vi "Initialize State Variables.vi"(8 "error in":errorcluster) -> (0 "error out":errorcluster, 2 "State Vars":T1)   [LabVIEW 2014, in "Waveform-Processing-Custom-Device Engine.lvlib"]
uses:
  Waveform-Processing-Custom-Device Engine.lvlib
  Types/StateVars.ctl
  Types/Async FIFOs.ctl
  Types/Async Settings.ctl
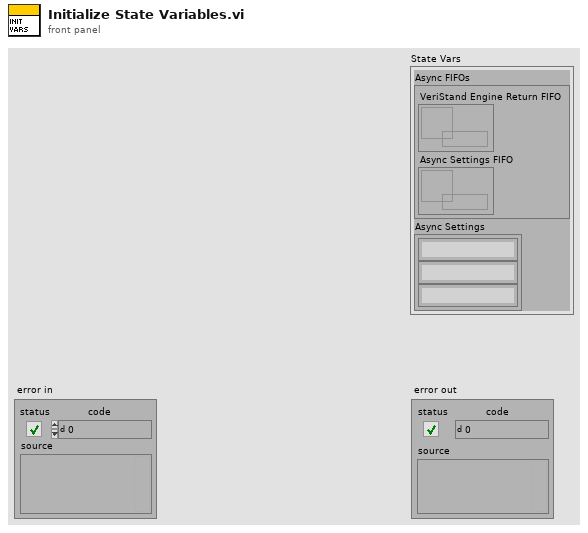
[diagram p1: front panel]
types:
  T1 = typedef "Waveform-Processing-Custom-Device Engine.lvlib/StateVars.ctl" = cluster{"Async FIFOs":T2, "Async Settings":T3}
  T2 = typedef "Async FIFOs.ctl" = cluster{"VeriStand Engine Return FIFO":refnum<k33>, "Async Settings FIFO":refnum<k33>}
  T3 = typedef "Waveform-Processing-Custom-Device Engine.lvlib/Async Settings.ctl" = cluster{string, string, string}
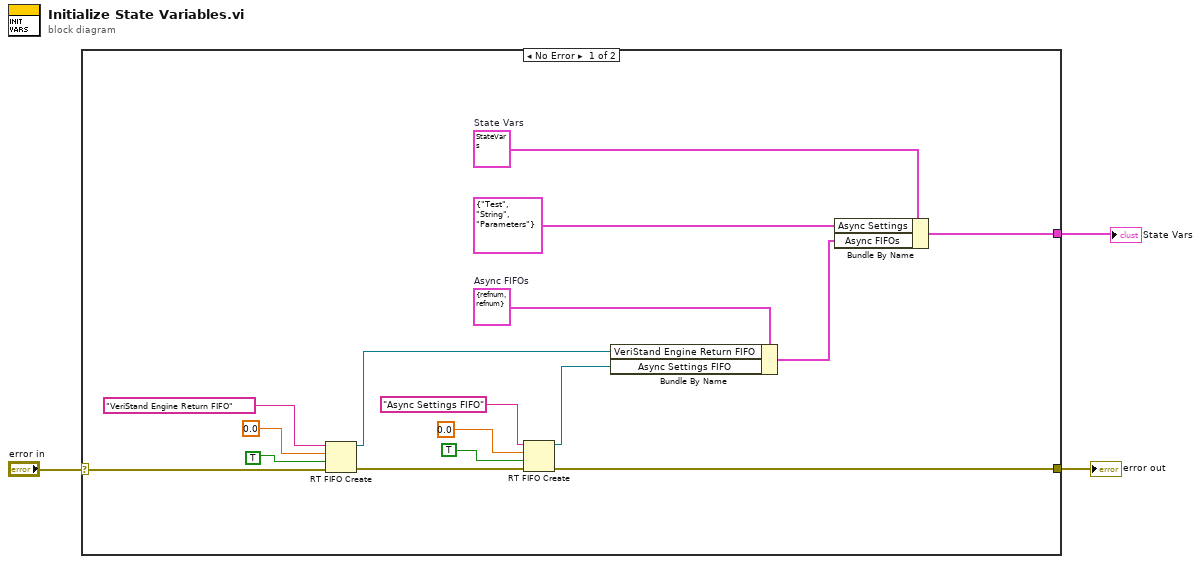
[diagram p0: block diagram]
diagram:
  n1 = case shown="No Error" "error in" {
    selector: "error in" -> [w19 w20]
    tunnel: [w13 w20] -> w2
    tunnel: [w4 _] -> w1
    frame No Error {
      w6 = T2 {"VeriStand Engine Return FIFO"=refnum, "Async Settings FIFO"=refnum}  # Async FIFOs
      w10 = T1 {"Async FIFOs"={"VeriStand Engine Return FIFO"=refnum, "Async Settings FIFO"=refnum}, "Async Settings"={"Test", "String", "Parameters"}}  # State Vars
      n2 = RT FIFO Create(0:"VeriStand Engine Return FIFO" ("name (unnamed)"), 1:0.0, 2:TRUE ("create if not found? (T)"), 3:w19) -> (8:w8:refnum<k33>, 11:w14:errorcluster)  [unwired: 4 in, 1 out]
      n3 = RT FIFO Create(0:"Async Settings FIFO" ("name (unnamed)"), 1:0.0, 2:TRUE ("create if not found? (T)"), 3:w14) -> (8:w7:refnum<k33>, 11:w13:errorcluster)  [unwired: 4 in, 1 out]
      n4 = Bundle By Name(cluster=w6, "VeriStand Engine Return FIFO"=w8, "Async Settings FIFO"=w7) -> (w5:T2)
      n5 = Bundle By Name(cluster=w10, "Async Settings"=T3 {"Test", "String", "Parameters"}, "Async FIFOs"=w5) -> (w4:T1)
    }
    frame Error {
    }
  }
  "error out" <- w2
  "State Vars" <- w1
